vi "FPGA - Delay.vi"(7 "Delay_ticks":u32, 8 "index":i32, 10 "Right Audio In":u64, 11 "Left Audio In":u64) -> (2 "Delayed Right":u64, 3 "Delayed Left":u64)   [LabVIEW 2014]
uses:
  <vilib>/rvi/Memory/Memory_Emulation/nirvimemoryFastEmulation.vi
  <vilib>/rvi/Memory/Memory_Emulation/nirvimemoryEmulation.vi
  <vilib>/rvi/Emulation/niFpgaEmulationIsFPGAContextNoSignature.vi
  <vilib>/rvi/DataTransferAndStorage/Container/Common/niFpgaContainerGetUniqueNameForEmu.vi
  <vilib>/rvi/Emulation/niFpgaProcessEmulError.vi
  <vilib>/rvi/Emulation/niFpgaSctlEmulationGetInTimedLoop.vi
  <vilib>/rvi/errors/nirviReportUnexpectedCaseInternalError (U32).vi
  <vilib>/rvi/DataTransferAndStorage/Container/XNode/niFpgaContainer.xnode
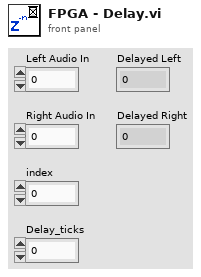
[diagram p1: front panel]
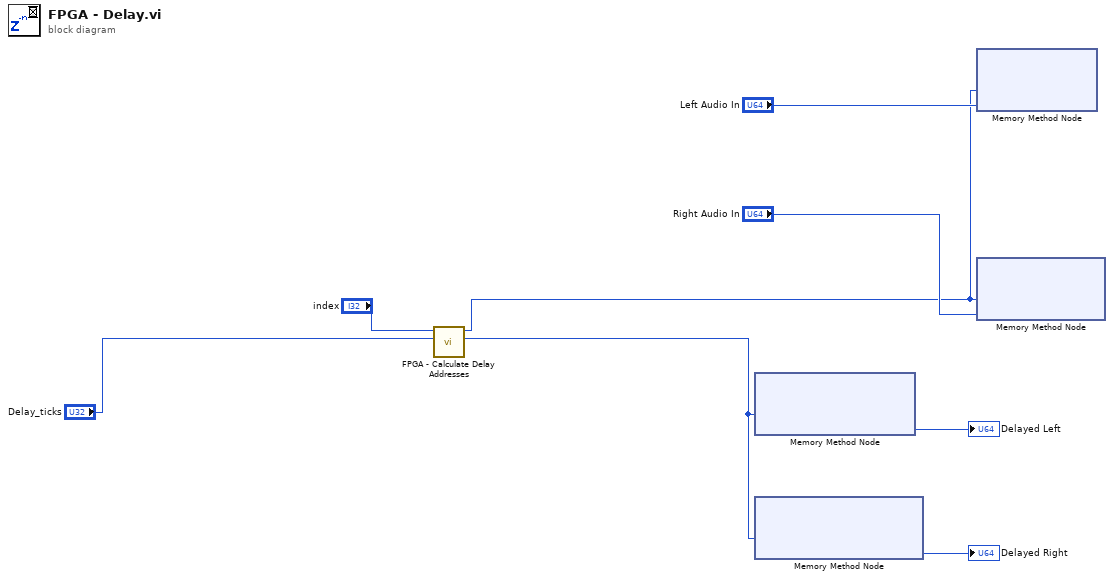
[diagram p0: block diagram]
diagram:
  n1 = call "FPGA - Calculate Delay Addresses.vi"("Delay_ticks"="Delay_ticks", "index"="index") -> ("Read Address"=w4:u32, "Write Address"=w3:u32)  [unwired: 8 in]
  n2 = xnode ("Memory Method Node")("Address"=w4) -> ("Data"=→"Delayed Left":u64)  [unwired: 1 in, 1 out]
  n3 = xnode ("Memory Method Node")("Address"=w4) -> ("Data"=→"Delayed Right":u64)  [unwired: 1 in, 1 out]
  n4 = xnode ("Memory Method Node")("Address"=w3, "Data"="Left Audio In") -> ()  [unwired: 1 in, 1 out]
  n5 = xnode ("Memory Method Node")("Address"=w3, "Data"="Right Audio In") -> ()  [unwired: 1 in, 1 out]
